vi "GreenOutCell.vi"(5 "ToModBus?":bool) -> (2 "Color":u32)   [LabVIEW 2012]
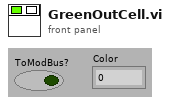
[diagram p1: front panel]
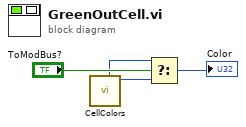
[diagram p0: block diagram]
diagram:
  n1 = call "CellColors.vi"() -> ("Normal"=w4:u32, "True"=w1:u32)  [unwired: 8 in, 2 out]
  n2 = Select(t=w1, s="ToModBus?", f=w4) -> (s? t:f=→"Color":u32)
